vi "VI Tree.vi"   [LabVIEW 2015, in "IT6700H.lvlib"]
doc: "This is the instrument driver for the <INSTRUMENT NAME>. The VI Tree displays all the user-callable VIs of the instrument driver in an organized table."
uses:
  <instrlib>/IT6700H/IT6700H.lvlib
panel:
  # "SEE DIAGRAM\nFOR VI TREE."
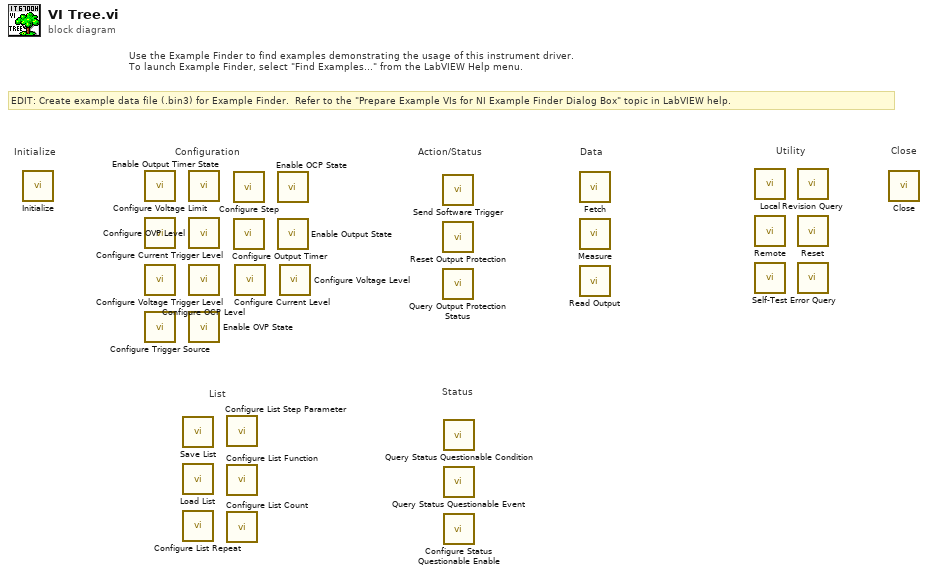
[diagram p0: block diagram]
diagram:
  # "Status"
  # "List"
  # "EDIT: Create example data file (.bin3) for Example Finder.  Refer to the \"Prepare Example VIs for NI Example Finder Dialog Box\" topic in LabVIEW help."
  # "Use the Example Finder to find examples demonstrating the usage of this instrument driver.\nTo launch Example Finder, select \"Find Examples...\" from the LabVIEW Help menu."
  # "Configuration"
  # "Utility"
  # "Data"
  # "Action/Status"
  # "Close"
  # "Initialize"
  n1 = call <instrlib>:"Initialize.vi"() -> ()  [unwired: 10 in, 2 out]
  n2 = call <instrlib>:"Configure Voltage Limit.vi"() -> ()  [unwired: 10 in, 2 out]
  n3 = call <instrlib>:"Configure Current Trigger Level.vi"() -> ()  [unwired: 10 in, 2 out]
  n4 = call <instrlib>:"Configure Voltage Trigger Level.vi"() -> ()  [unwired: 10 in, 2 out]
  n5 = call <instrlib>:"Configure Trigger Source.vi"() -> ()  [unwired: 10 in, 2 out]
  n6 = call <instrlib>:"Save List.vi"() -> ()  [unwired: 10 in, 2 out]
  n7 = call <instrlib>:"Load List.vi"() -> ()  [unwired: 10 in, 2 out]
  n8 = call <instrlib>:"Configure List Repeat.vi"() -> ()  [unwired: 10 in, 2 out]
  n9 = call <instrlib>:"Enable Output Timer State.vi"() -> ()  [unwired: 10 in, 2 out]
  n10 = call <instrlib>:"Configure OVP Level.vi"() -> ()  [unwired: 10 in, 2 out]
  n11 = call <instrlib>:"Configure OCP Level.vi"() -> ()  [unwired: 10 in, 2 out]
  n12 = call <instrlib>:"Enable OVP State.vi"() -> ()  [unwired: 10 in, 2 out]
  n13 = call <instrlib>:"Configure List Step Parameter.vi"() -> ()  [unwired: 10 in, 2 out]
  n14 = call <instrlib>:"Configure List Function.vi"() -> ()  [unwired: 10 in, 2 out]
  n15 = call <instrlib>:"Configure List Count.vi"() -> ()  [unwired: 10 in, 2 out]
  n16 = call <instrlib>:"Configure Step.vi"() -> ()  [unwired: 10 in, 2 out]
  n17 = call <instrlib>:"Configure Output Timer.vi"() -> ()  [unwired: 10 in, 2 out]
  n18 = call <instrlib>:"Configure Current Level.vi"() -> ()  [unwired: 10 in, 2 out]
  n19 = call <instrlib>:"Enable OCP State.vi"() -> ()  [unwired: 10 in, 2 out]
  n20 = call <instrlib>:"Enable Output State.vi"() -> ()  [unwired: 9 in, 2 out]
  n21 = call <instrlib>:"Configure Voltage Level.vi"() -> ()  [unwired: 10 in, 2 out]
  n22 = call <instrlib>:"Send Software Trigger.vi"() -> ()  [unwired: 10 in, 2 out]
  n23 = call <instrlib>:"Reset Output Protection.vi"() -> ()  [unwired: 10 in, 2 out]
  n24 = call <instrlib>:"Query Output Protection Status.vi"() -> ()  [unwired: 8 in, 4 out]
  n25 = call <instrlib>:"Query Status Questionable Condition.vi"() -> ()  [unwired: 9 in, 3 out]
  n26 = call <instrlib>:"Query Status Questionable Event.vi"() -> ()  [unwired: 9 in, 3 out]
  n27 = call <instrlib>:"Configure Status Questionable Enable.vi"() -> ()  [unwired: 10 in, 2 out]
  n28 = call <instrlib>:"Fetch.vi"() -> ()  [unwired: 9 in, 3 out]
  n29 = call <instrlib>:"Measure.vi"() -> ()  [unwired: 9 in, 3 out]
  n30 = call <instrlib>:"Read Output.vi"() -> ()  [unwired: 8 in, 4 out]
  n31 = call <instrlib>:"Local.vi"() -> ()  [unwired: 10 in, 2 out]
  n32 = call <instrlib>:"Remote.vi"() -> ()  [unwired: 10 in, 2 out]
  n33 = call <instrlib>:"Self-Test.vi"() -> ()  [unwired: 8 in, 4 out]
  n34 = call <instrlib>:"Revision Query.vi"() -> ()  [unwired: 8 in, 4 out]
  n35 = call <instrlib>:"Reset.vi"() -> ()  [unwired: 10 in, 2 out]
  n36 = call <instrlib>:"Error Query.vi"() -> ()  [unwired: 8 in, 4 out]
  n37 = call <instrlib>:"Close.vi"() -> ()  [unwired: 11 in, 1 out]
